vi "Sequence Raffle.vi"(2 "Number of Raffles":i32, 3 "Game Data In":T1) -> (1 "Game Data Out":T1)   [LabVIEW 2019]
uses:
  Controls/Game Data.ctl
  <vilib>/numeric/Random Number (Range) U64.vi
  <vilib>/numeric/sub_Random U32.vi
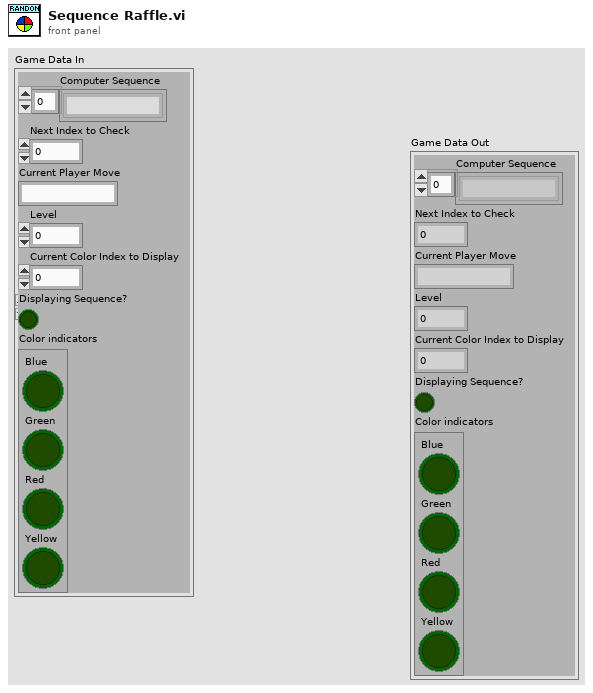
[diagram p1: front panel]
types:
  T1 = typedef "Game Data.ctl" = cluster{"Computer Sequence":string[], "Next Index to Check":i32, "Current Player Move":string, "Level":i32, "Current Color Index to Display":i32, "Displaying Sequence?":bool, "Color indicators":cluster{"Blue":bool, "Green":bool, "Red":bool, "Yellow":bool}}
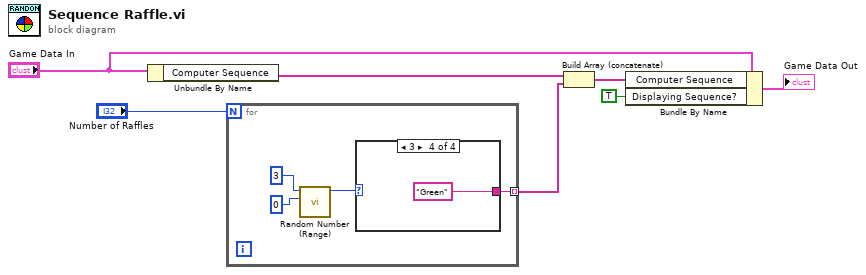
[diagram p0: block diagram]
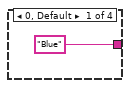
[diagram p2: hidden frame]
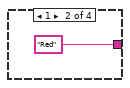
[diagram p3: hidden frame]
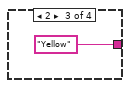
[diagram p4: hidden frame]
diagram:
  n1 = Unbundle By Name("Game Data In") -> ("Computer Sequence"=w6:string[])
  n2 = for {
    N: "Number of Raffles" -> [_]
    tunnel: [w8] -> w5 mode=indexing
    n3 = call-poly <vilib>:"Random Number (Range).vi"("lower bound (0)"=u64 0, "upper bound (100)"=u64 3) -> ("number"=w9:u64)  [unwired: 9 in]
    n4 = case shown="3" w9 {
      tunnel: ["Blue" "Red" "Yellow" "Green"] -> w8
      frame 0, Default {
      }
      frame 1 {
      }
      frame 2 {
      }
      frame 3 {
      }
    }
  }
  n5 = Build Array (concatenate)(w6, w5) -> (w3:string[])
  n6 = Bundle By Name(cluster="Game Data In", "Computer Sequence"=w3, "Displaying Sequence?"=TRUE) -> (→"Game Data Out":T1)
